vi "Compare.vi"(10 "Top Future":refnum<class "Future.lvclass">, 11 "Future in":refnum<class "Future.lvclass">) -> (3 "Boolean":bool)   [LabVIEW 2017, in "Promise Future.lvlib" / "Future.lvclass"]
uses:
  Future.lvclass
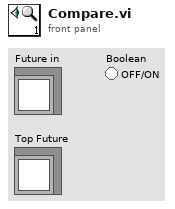
[diagram p1: front panel]
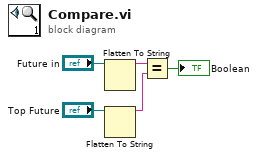
[diagram p0: block diagram]
diagram:
  n1 = Flatten To String(anything="Future in") -> (data string=w2:string)  [unwired: 3 in, 2 out]
  n2 = Flatten To String(anything="Top Future") -> (data string=w1:string)  [unwired: 3 in, 2 out]
  n3 = Equal?(x=w2, y=w1) -> (x = y?=→"Boolean":bool)
